vi "Exemple_Kernel_App_SkewedChi2Sampler.vi"() -> ()   [LabVIEW 2020]
uses:
  Objet/6 - Datasets Transformation/6.7 - Kernel Approximation/SkewedChi2Sampler/SkewedChi2Sampler.lvclass
panel:
  in  "SkewedChi2Sampler":T1={"skewedness"=1.0, "n_components"=100, "random_state"=-1} {"random_state" min=-1}
  in  "y":string[][](array[string])
  out "error out":errorcluster caption="sortie d'erreur"
  out "Data":T2
  in  "error in":errorcluster caption="entrée d'erreur"
  in  "X":string[][](array[string])=[["0", "0"], ["1", "1"], ["1", "0"], ["0", "1"]]
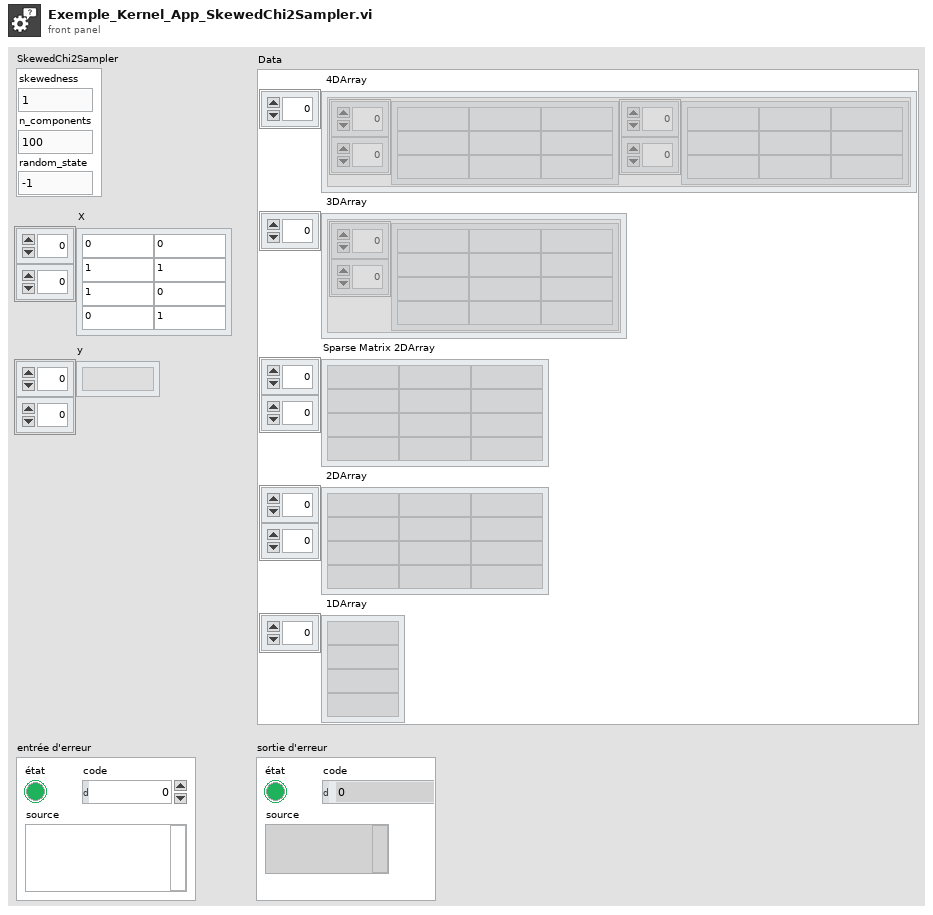
[diagram p1: front panel]
types:
  T1 = cluster{"skewedness":dbl, "n_components":i32, "random_state":i32}
  T2 = cluster{" 4DArray":cluster{"1":string[][], "2":string[][]}[], " 3DArray":cluster{"Tableau":string[][]}[], "Sparse Matrix 2DArray":string[][], " 2DArray":string[][], " 1DArray":string[]}
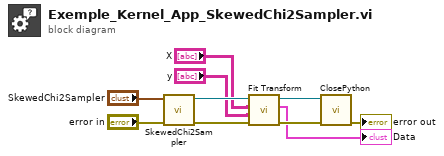
[diagram p0: block diagram]
diagram:
  n1 = call "SkewedChi2Sampler.vi"("error in"="error in", "SkewedChi2Sampler"="SkewedChi2Sampler") -> ("error out"=w4:errorcluster, "SkewedChi2Sampler.lvclass"=w7:refnum<class "SkewedChi2Sampler.lvclass">)  [unwired: 8 in]
  n2 = call-dynamic "Fit Transform.vi"("error in (no error)"=w4, "y"="y", "X"="X", "SkewedChi2Sampler.lvclass"=w7) -> ("error in (no error)"=w3:errorcluster, "Data"=→"Data":T2, "SkewedChi2Sampler.lvclass"=w2:refnum<class "SkewedChi2Sampler.lvclass">)  [unwired: 5 in]
  n3 = call-dynamic "ClosePython.vi"("error in (no error)"=w3, "Scikit-learn en entrée"=w2) -> ("error out"=→"error out":errorcluster)  [unwired: 8 in, 1 out]
